vi "LV21_1_1.vi"() -> ()   [LabVIEW 2021]
panel:
  out "Execution Time Total":dbl
  out "Execution Time Part 2":dbl
  out "Execution Time Part 1":dbl
  out "Part 1 RESULT":i32
  out "Part 2 RESULT":i32
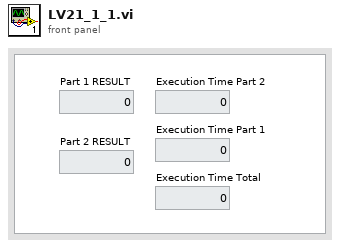
[diagram p1: front panel]
types:
  T1 = map{i32, cluster{"Elv Number":i32, "Number of Items":i32}}
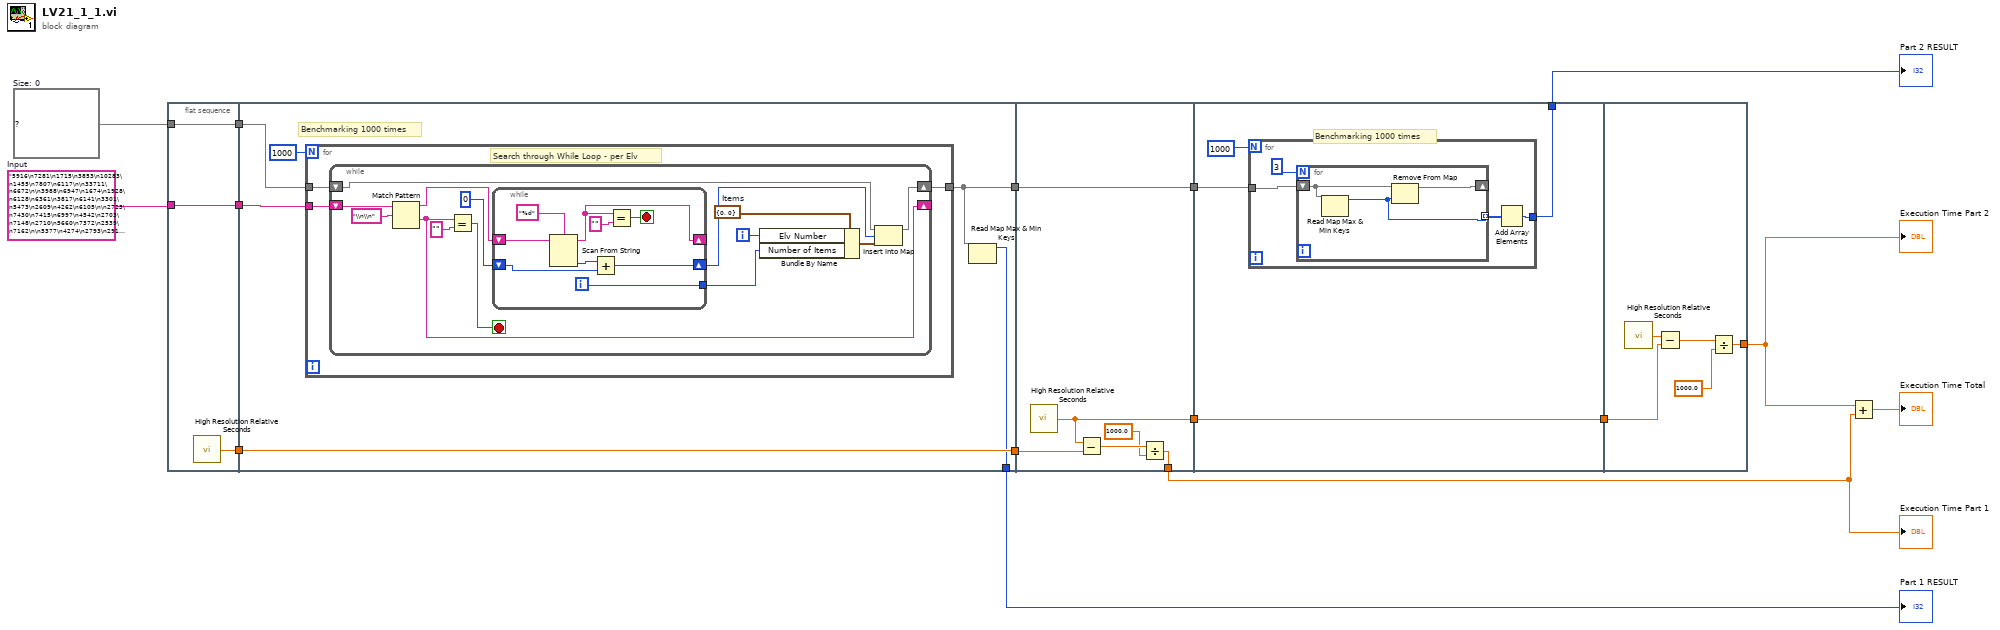
[diagram p0: block diagram]
diagram:
  w14 = T1 {}  # Size: 0
  w15 = "5916\n7281\n1715\n3853\n10283\n1455\n7807\n6117\n\n33711\n6672\n\n3988\n6947\n1674\n1928\n6128\n6361\n3817\n6141\n3301\n5473\n2609\n4262\n6105\n\n2725\n7430\n7415\n6997\n4542\n2703\n7148\n2710\n5660\n7372\n2539\n7162\n\n5377\n4274\n2793\n2911\n2113\n1077\n4115\n5871\n1079\n4336\n4894\n2088\n5408\n5535\n1982\n\n3270\n1347\n4884\n2986\n6067\n5567\n5093\n4421\n2772\n4935\n6153\n1235\n3824\n6460\n\n4131\n5183\n5329\n8021\n6096\n6053\n4352\n2016\n5055\n3031\n3379\n\n1846\n3964\n16169\n10061\n16400\n\n1519\n5378\n6590\n6782\n7072\n4011\n6581\n5871\n6112\n6836\n\n3894\n5621\n6342\n6746\n1955\n3348\n5651\n1468\n7232\n3240\n3435\n4566\n\n8079\n4170\n5034\n\n7439\n1078\n4537\n7020\n2013\n2796\n1627\n1171\n3472\n2611\n3701\n1570..."  # Input
  n1 = flat-sequence {
    tunnel: w14 -> [w17]
    tunnel: w15 -> [w18]
    tunnel: [w18] -> w13
    tunnel: [w17] -> w12
    tunnel: [w16] -> w8
    tunnel: w13 -> [w24]
    tunnel: w12 -> [w23]
    tunnel: [w22] -> w11
    tunnel: [w21] -> w9
    tunnel: w8 -> [w21]
    tunnel: [w20] -> w5
    tunnel: w11 -> [w56]
    tunnel: [w56] -> w10
    tunnel: w9 -> [w54]
    tunnel: [w51] -> w6
    tunnel: [w52] -> w2
    tunnel: w10 -> [w60]
    tunnel: [w59] -> w7
    tunnel: w6 -> [w59]
    tunnel: [w58] -> w4
    tunnel: w7 -> [w71]
    tunnel: [w69] -> w3
    frame #0 {
      n2 = call <vilib>:"High Resolution Relative Seconds.vi"() -> ("relative seconds"=w16:dbl)
    }
    frame #1 {
      # "Benchmarking 1000 times"
      n3 = for {
        N: 1000 -> [_]
        tunnel: w24 -> [w27]
        tunnel: w23 -> [w26]
        tunnel: [w25] -> w22
        # "Search through While Loop - per Elv"
        n4 = while {
          shift-right: [w30] -> _
          shift-left: w27 -> [w40]
          shift-right: [w33] -> w25
          shift-left: w26 -> [w35]
          i -> [w28]
          stop <- w31 stop-if-true
          w37 = cluster{"Elv Number":i32, "Number of Items":i32} {"Elv Number"=0, "Number of Items"=0}  # Items
          n5 = Match Pattern(string=w40, regular expression="\\n\\n") -> (before substring=w39:string, after substring=w30:string)  [unwired: 1 in, 2 out]
          n6 = Equal?(x=w30, y="") -> (x = y?=w31:bool)
          n7 = while {
            shift-right: [w46] -> w29
            shift-left: 0 ("output 1") -> [w44]
            tunnel: [w43] -> w36
            shift-right: [w42] -> _
            shift-left: w39 -> [w50]
            i -> [w43]
            stop <- w47 stop-if-true
            n8 = Scan From String(format string="%d", input string=w50) -> (remaining string=w42:string, output 1=w45:i32)  [unwired: 3 in, 2 out]
            n9 = Add(x=w45, y=w44) -> (x+y=w46:i32)
            n10 = Equal?(x=w42, y="") -> (x = y?=w47:bool)
          }
          n11 = Bundle By Name(cluster=w37, "Elv Number"=w28, "Number of Items"=w36) -> (w34:cluster{"Elv Number":i32, "Number of Items":i32})
          n12 = Insert Into Map(map in=w35, key=w29, value=w34) -> (map out=w33:T1)  [unwired: 2 out]
        }
      }
      n13 = Read Map Max & Min Keys(11:w22) -> (3:w20:i32)  [unwired: 1 out]
    }
    frame #2 {
      n14 = call <vilib>:"High Resolution Relative Seconds.vi"() -> ("relative seconds"=w51:dbl)
      n15 = Subtract(x=w51, y=w54) -> (x-y=w55:dbl)
      n16 = Divide(x=w55, y=1000.0) -> (x/y=w52:dbl)
    }
    frame #3 {
      # "Benchmarking 1000 times"
      n17 = for {
        N: 1000 -> [_]
        tunnel: w60 -> [w62]
        tunnel: [w61] -> w58
        n18 = for {
          N: 3 -> [_]
          tunnel: [w65] -> w64 mode=indexing
          shift-right: [w66] -> _
          shift-left: w62 -> [w67]
          n19 = Read Map Max & Min Keys(11:w67) -> (3:w65:i32)  [unwired: 1 out]
          n20 = Remove From Map(10:w65, 11:w67) -> (3:w66:T1)  [unwired: 2 out]
        }
        n21 = Add Array Elements(numeric array=w64) -> (sum=w61:i32)
      }
    }
    frame #4 {
      n22 = call <vilib>:"High Resolution Relative Seconds.vi"() -> ("relative seconds"=w72:dbl)
      n23 = Subtract(x=w72, y=w71) -> (x-y=w70:dbl)
      n24 = Divide(x=w70, y=1000.0) -> (x/y=w69:dbl)
    }
  }
  n25 = Add(x=w3, y=w2) -> (x+y=→"Execution Time Total":dbl)
  "Execution Time Part 1" <- w2
  "Execution Time Part 2" <- w3
  "Part 1 RESULT" <- w5
  "Part 2 RESULT" <- w4
